vi "Log_Reference_Velocity.vi"(1 "Measured Velocity":dbl) -> ()   [LabVIEW 2022 SP3]
uses:
  Controls/Server_Comms.ctl
  Controls/Post_Process.ctl
  File/Setup_Filetype.ctl
  Globals/Meas_global.vi
  Globals/Preference_global.vi
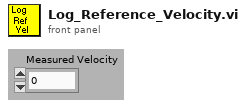
[diagram p1: front panel]
types:
  T1 = typedef "Post_Process.ctl" = enum16{"Take New Data", "Post Process Raw Data File"}
  T2 = typedef "Server_Comms.ctl" = enum16{"Do Not Link To Server", "Server Link Healthy"}
  T3 = typedef "Setup_Filetype.ctl" = enum16{"Measurement Setups", "Calibration Setups", "General", "Results File Plotter Setups", "Speed Calib Tweaks"}
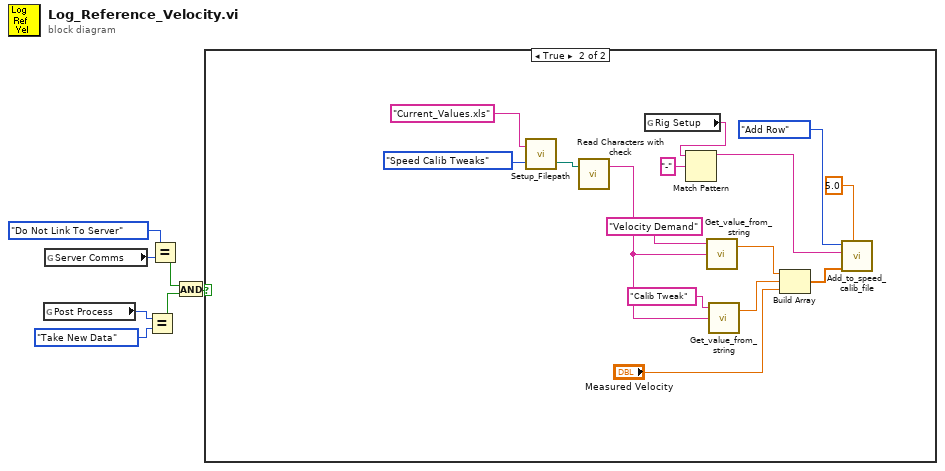
[diagram p0: block diagram]
diagram:
  n1 = global read "Meas_global.vi" "Post Process"() -> (w6:T1)
  n2 = global read "Preference_global.vi" "Server Comms"() -> (w5:T2)
  n3 = Equal?(x=w6, y=Post_Process."Take New Data" ("Post Process")) -> (x = y?=w3:bool)
  n4 = Equal?(x=Server_Comms."Do Not Link To Server" ("Server Comms"), y=w5) -> (x = y?=w2:bool)
  n5 = And(x=w2, y=w3) -> (x .and. y?=w1:bool)
  n6 = case shown="True" w1 {
    frame False {
    }
    frame True {
      n7 = call "Setup_Filepath.vi"("Setup File Type"=Setup_Filetype."Speed Calib Tweaks", "Filename in"="Current_Values.xls" ("name or relative path")) -> ("Filename Out"=w9:path)  [unwired: 1 out]
      n8 = call "Read Characters with check.vi"("file (use dialog)"=w9) -> ("Read String"=w8:string)  [unwired: 1 in, 1 out]
      n9 = global read "Preference_global.vi" "Rig Setup"() -> (w15:string)
      n10 = Match Pattern(string=w15, regular expression="-") -> (before substring=w13:string)  [unwired: 4 out]
      n11 = call "Get_value_from_string.vi"("Input string"=w8, "Variable name"="Velocity Demand") -> ("Value"=w20:dbl)  [unwired: 1 in, 1 out]
      n12 = call "Get_value_from_string.vi"("Input string"=w8, "Variable name"="Calib Tweak") -> ("Value"=w19:dbl)  [unwired: 1 in, 1 out]
      n13 = Build Array(w20, w19, "Measured Velocity") -> (w17:dbl[])
      n14 = call "Add_to_speed_calib_file.vi"("Max Velocity"=5.0, "New Row"=w17, "Rig Name"=w13, "Mode"=enum16{"Add Row", "Get Error Value"}."Add Row") -> ()  [unwired: 1 in, 3 out]
    }
  }
